vi "Ramp SUBVI.vi"   [LabVIEW 2011]
types:
  T1 = cluster{"Digital Input [1-16][0]":bool, "Digital Input [1-16][1]":bool, "Digital Input [1-16][2]":bool, "Digital Input [1-16][3]":bool, "Digital Input [1-16][4]":bool, "Digital Input [1-16][5]":bool, "Digital Input [1-16][6]":bool, "Digital Input [1-16][7]":bool, "Digital Input [1-16][8]":bool, "Digital Input [1-16][9]":bool, "Digital Input [1-16][10]":bool, "Digital Input [1-16][11]":bool, "Digital Input [1-16][12]":bool, "Digital Input [1-16][13]":bool, "Digital Input [1-16][14]":bool, "Digital Input [1-16][15]":bool}
  T2 = typedef "WPI_DigitalInputDevRef.ctl" = cluster{"DevStatus":errorcluster, "DIO Channel":T3, "Digital Module":T4}
  T3 = typedef "FPGA_DIOChannel.ctl" = enum8{"DIO 1", "DIO 2", "DIO 3", "DIO 4", "DIO 5", "DIO 6", "DIO 7", "DIO 8", "DIO 9", "DIO 10", "DIO 11", "DIO 12", "DIO 13", "DIO 14", "Invalid"}
  T4 = typedef "FPGA_TypedefDigitalModule.ctl" = enum16{"Digital Module 1", "Digital Module 2"}
  T5 = typedef "WPI_MotorControlDeviceRef.ctl" = cluster{"DeviceStatus":errorcluster, "Type":enum16{"PWM", "CAN"}, "PWM":cluster{"Digital Module":T4, "PWM Channel":T6, "DeadBand":T7}, "CAN":cluster{"Device Number":u8, "Control Mode":T8, "Semaphore":T9, "Max Vout":dbl}, "Invert":bool, "TransformRef":T10, "InvTransformRef":T10}
  T6 = typedef "FPGA_DIOPWMChannel.ctl" = enum8{"PWM 1", "PWM 2", "PWM 3", "PWM 4", "PWM 5", "PWM 6", "PWM 7", "PWM 8", "PWM 9", "PWM 10", "Invalid"}
  T7 = typedef "WPI_PWMDeadband.ctl" = cluster{"Name":string, "maxPositivePwm":i32, "minPositivePwm":i32, "centerPwm":i32, "maxNegativePwm":i32, "minNegativePwm":i32, "angularRange":u16}
  T8 = typedef "WPI_CANJaguar_ControlMode.ctl" = enum8{"Percent VBus", "Current", "Speed", "Position", "Voltage"}
  T9 = typedef "Semaphore RefNum" = refnum<k1>
  T10 = typedef "WPI_PWMTransform_ConPane.ctl" = refnum<vi>
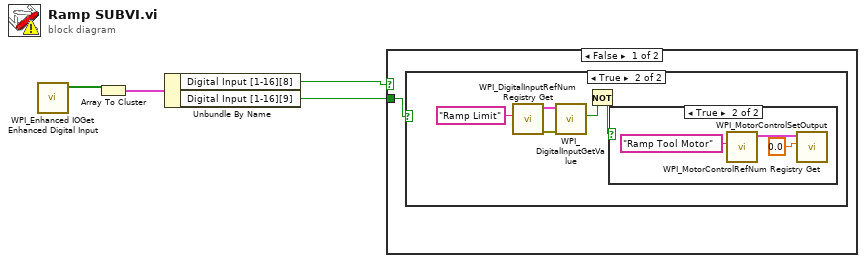
[diagram p0: block diagram]
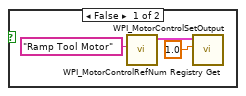
[diagram p3: hidden frame]
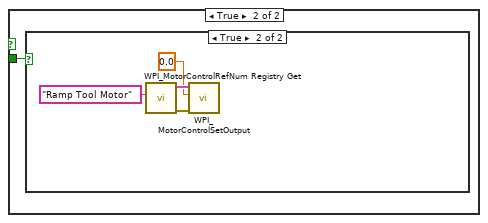
[diagram p4: hidden frame]
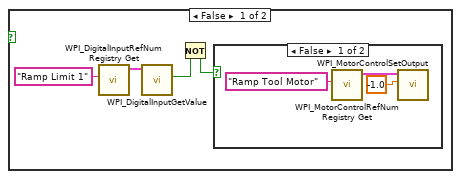
[diagram p5: hidden frame]
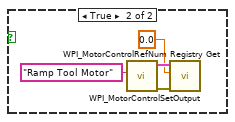
[diagram p6: hidden frame]
diagram:
  n1 = call <vilib>:"WPI_Enhanced IOGet Enhanced Digital Input.vi"() -> ("Digital Input [1-16]"=w3:bool[])  [unwired: 10 in, 1 out]
  n2 = Array To Cluster(array=w3) -> (cluster=w4:T1)
  n3 = Unbundle By Name(w4) -> ("Digital Input [1-16][8]"=w2:bool, "Digital Input [1-16][9]"=w1:bool)
  n4 = case shown="False" w2 {
    tunnel: w1 -> [w5 w17]
    frame False {
      n5 = case shown="True" w5 {
        frame False {
        }
        frame True {
          n6 = call <vilib>:"WPI_DigitalInputRefNum Registry Get.vi"("refnum name"="Ramp Limit") -> ("error out"=w10:errorcluster, "DigitalInputDevRef"=w9:T2)  [unwired: 9 in]
          n7 = call <vilib>:"WPI_DigitalInputGetValue.vi"("error in (no error)"=w10, "DigitalInputDevRef"=w9) -> ("Value"=w7:bool)  [unwired: 7 in, 2 out]
          n8 = Not(x=w7) -> (.not. x?=w6:bool)
          n9 = case shown="True" w6 {
            frame False {
              n10 = call <vilib>:"WPI_MotorControlRefNum Registry Get.vi"("refnum name"="Ramp Tool Motor") -> ("MotorControlDevRef"=w13:T5)  [unwired: 9 in, 1 out]
              n11 = call <vilib>:"WPI_MotorControlSetOutput.vi"("Output"=1.0, "MotorControlDevRef"=w13) -> ()  [unwired: 8 in, 2 out]
            }
            frame True {
              n12 = call <vilib>:"WPI_MotorControlRefNum Registry Get.vi"("refnum name"="Ramp Tool Motor") -> ("MotorControlDevRef"=w14:T5)  [unwired: 9 in, 1 out]
              n13 = call <vilib>:"WPI_MotorControlSetOutput.vi"("Output"=0.0, "MotorControlDevRef"=w14) -> ()  [unwired: 8 in, 2 out]
            }
          }
        }
      }
    }
    frame True {
      n14 = case shown="True" w17 {
        frame False {
          n15 = call <vilib>:"WPI_DigitalInputRefNum Registry Get.vi"("refnum name"="Ramp Limit 1") -> ("DigitalInputDevRef"=w20:T2)  [unwired: 9 in, 1 out]
          n16 = call <vilib>:"WPI_DigitalInputGetValue.vi"("DigitalInputDevRef"=w20) -> ("Value"=w19:bool)  [unwired: 8 in, 2 out]
          n17 = Not(x=w19) -> (.not. x?=w18:bool)
          n18 = case shown="False" w18 {
            frame False {
              n19 = call <vilib>:"WPI_MotorControlRefNum Registry Get.vi"("refnum name"="Ramp Tool Motor") -> ("MotorControlDevRef"=w24:T5)  [unwired: 9 in, 1 out]
              n20 = call <vilib>:"WPI_MotorControlSetOutput.vi"("Output"=-1.0, "MotorControlDevRef"=w24) -> ()  [unwired: 8 in, 2 out]
            }
            frame True {
              n21 = call <vilib>:"WPI_MotorControlRefNum Registry Get.vi"("refnum name"="Ramp Tool Motor") -> ("error out"=w27:errorcluster, "MotorControlDevRef"=w28:T5)  [unwired: 9 in]
              n22 = call <vilib>:"WPI_MotorControlSetOutput.vi"("error in (no error)"=w27, "Output"=0.0, "MotorControlDevRef"=w28) -> ()  [unwired: 7 in, 2 out]
            }
          }
        }
        frame True {
          n23 = call <vilib>:"WPI_MotorControlRefNum Registry Get.vi"("refnum name"="Ramp Tool Motor") -> ("error out"=w31:errorcluster, "MotorControlDevRef"=w32:T5)  [unwired: 9 in]
          n24 = call <vilib>:"WPI_MotorControlSetOutput.vi"("error in (no error)"=w31, "Output"=0.0, "MotorControlDevRef"=w32) -> ()  [unwired: 7 in, 2 out]
        }
      }
    }
  }
